vi "Lake Shore 331 Temperature Controller v2.vi"(1 "Loop (0: 1)":u16(ring) items=["1", "2"], 2 "Gain (P)":dbl=50.0 min=0.0 max=1000.0 step=0.1 format="%.1f", 3 "Reset (I)":dbl=50.0 min=0.0 max=1000.0 step=0.1 format="%.1f", 4 "Rate (D)":dbl=100.0 min=0.0 max=200.0 step=1.0, 7 "Manual Output":dbl min=0.0 max=100.0 step=0.001 format="%.3f", 9 "Heater Range (0: Off)":u16(ring)=3 items=["Off", "Low (0.5W)", "Med (5W)", "High (50W)"]) -> (16 "Sensor A":dbl=314.34 min=0.0 max=1645.0 step=1e-05 format="%.5f", 18 "Heater Output":dbl(slide)=100.0 min=0.0 max=100.0 step=0.01 scale=0.0..100.0 scale format="%.1f")   [LabVIEW 2015]
doc: "This VI was designed to demonstrate typical usage of sub vi's containing the more common 331 functions.\n\nThis example configures the loop and setpoint of the instrument, allows for a delay, and then reads sensor and heater output data. The user is given the option of just reading data and not configuring the instrument."
uses:
  <vilib>/Utility/file.llb/Write Delimited Spreadsheet (DBL).vi
  <instrlib>/Lake Shore Cryotronics 331/Lake Shore Cryotronics 331.lvlib
panel:
  in  "Reset":bool
  out "XY Graph":cluster{dbl[], dbl[]}[](graph)=[{array[256 elements], [302.68, 302.68, 302.68, 302.68, 302.68, 302.68, 302.68, 302.68, 302.68, 302.68, 302.68, 302.68, 302.68, 302.68, 302.68, 302.68, 302.68, 302.68, 302.68, 302.68, 302.68, 302.68, 302.68, 302.68, 302.68, 302.68, 302.68, 302.68, 302.68, 302.68, 302.68, 302.68, 302.68, 302.68, 302.68, 302.68, 302.68, 302.68, 302.68, 302.68, 302.68, 302.68, 302.68, 302.68, 302.68, 302.68, 302.68, 302.68, 302.68, 302.68, 302.68, 302.68, 302.68, 302.68, 302.68, 302.68, 302.69, 302.69, 302.69, 302.69, 302.69, 302.69, 302.69, 302.69, 302.7, 302.7, 302.7, 302.7, 302.71, 302.71, 302.72, 302.72, 302.73, 302.73, 302.74, 302.75, 302.76, 302.76, 302.77, 302.78, 302.79, 302.8, 302.82, 302.83, 302.84, 302.85, 302.87, 302.88, 302.9, 302.92, 302.93, 302.95, 302.97, 302.99, 303.01, 303.03, 303.05, 303.08, 303.1, 303.12, 303.15, 303.17, 303.2, 303.23, 303.26, 303.29, 303.32, 303.35, 303.38, 303.41, 303.44, 303.48, 303.51, 303.55, 303.59, 303.62, 303.66, 303.7, 303.74, 303.78, 303.82, 303.86, 303.91, 303.95, 303.99, 304.04, 304.08, 304.13, 304.18, 304.22, 304.27, 304.32, 304.37, 304.42, 304.47, 304.53, 304.58, 304.63, 304.69, 304.74, 304.8, 304.85, 304.91, 304.97, 305.03, 305.09, 305.15, 305.21, 305.27, 305.33, 305.39, 305.45, 305.52, 305.58, 305.64, 305.71, 305.77, 305.84, 305.91, 305.97, 306.04, 306.11, 306.18, 306.25, 306.32, 306.39, 306.46, 306.53, 306.6, 306.67, 306.75, 306.82, 306.89, 306.97, 307.04, 307.12, 307.19, 307.27, 307.34, 307.42, 307.5, 307.58, 307.65, 307.73, 307.81, 307.89, 307.97, 308.05, 308.13, 308.21, 308.3, 308.38, 308.46, 308.54, 308.63, 308.71, 308.79, 308.88, 308.96, 309.05, 309.13, 309.22, 309.3, 309.39, 309.48, 309.56, 309.65, 309.74, 309.82, 309.91, 310.0, 310.09, 310.18, 310.27, 310.36, 310.45, 310.54, 310.63, 310.72, 310.81, 310.9, 310.99, 311.08, 311.18, 311.27, 311.36, 311.45, 311.55, 311.64, 311.73, 311.83, 311.92, 312.02, 312.11, 312.2, 312.3, 312.4, 312.49, 312.59, 312.68, 312.78, 312.88, 312.97, 313.07, 313.17, 313.26, 313.36, 313.46, 313.55, 313.65, 313.75, 313.85, 313.95, 314.04, 314.14, 314.24]}, {array[256 elements], [302.29, 302.29, 302.29, 302.29, 302.29, 302.29, 302.29, 302.29, 302.29, 302.29, 302.29, 302.29, 302.29, 302.29, 302.29, 302.29, 302.29, 302.29, 302.29, 302.29, 302.29, 302.29, 302.29, 302.29, 302.29, 302.29, 302.29, 302.29, 302.29, 302.29, 302.29, 302.29, 302.32, 302.31, 302.31, 302.34, 302.42, 302.56, 302.76, 303.03, 303.34, 303.7, 304.1, 304.52, 304.97, 305.44, 305.93, 306.42, 306.92, 307.42, 307.93, 308.43, 308.93, 309.43, 309.92, 310.41, 310.89, 311.37, 311.83, 312.29, 312.75, 313.19, 313.63, 314.06, 314.48, 314.89, 315.29, 315.69, 316.08, 316.47, 316.84, 317.21, 317.57, 317.93, 318.28, 318.63, 318.96, 319.3, 319.62, 319.94, 320.26, 320.57, 320.87, 321.17, 321.46, 321.75, 322.04, 322.32, 322.6, 322.87, 323.14, 323.41, 323.67, 323.93, 324.18, 324.43, 324.69, 324.93, 325.18, 325.42, 325.66, 325.9, 326.13, 326.36, 326.59, 326.82, 327.04, 327.27, 327.49, 327.71, 327.92, 328.14, 328.35, 328.56, 328.77, 328.98, 329.19, 329.39, 329.6, 329.8, 330.0, 330.2, 330.4, 330.59, 330.79, 330.98, 331.17, 331.37, 331.56, 331.74, 331.93, 332.12, 332.3, 332.49, 332.67, 332.86, 333.04, 333.22, 333.4, 333.58, 333.75, 333.93, 334.11, 334.29, 334.46, 334.64, 334.81, 334.99, 335.16, 335.33, 335.5, 335.67, 335.84, 336.01, 336.18, 336.35, 336.52, 336.69, 336.85, 337.02, 337.18, 337.35, 337.51, 337.68, 337.84, 338.0, 338.17, 338.33, 338.49, 338.65, 338.81, 338.97, 339.13, 339.29, 339.45, 339.61, 339.77, 339.92, 340.08, 340.23, 340.39, 340.54, 340.7, 340.86, 341.01, 341.17, 341.32, 341.47, 341.63, 341.78, 341.93, 342.09, 342.24, 342.39, 342.54, 342.69, 342.85, 343.0, 343.15, 343.27, 343.42, 343.57, 343.72, 343.86, 344.01, 344.16, 344.31, 344.46, 344.61, 344.75, 344.9, 345.05, 345.19, 345.34, 345.49, 345.63, 345.78, 345.92, 346.07, 346.21, 346.36, 346.5, 346.64, 346.78, 346.93, 347.07, 347.21, 347.35, 347.5, 347.64, 347.78, 347.92, 348.06, 348.2, 348.34, 348.48, 348.62, 348.76, 348.9, 349.04, 349.18, 349.32, 349.46, 349.6, 349.74, 349.88, 350.02, 350.15, 350.29, 350.43, 350.57, 350.7, 350.84, 350.98, 351.11, 351.25]}]
  in  "Save":bool
  out "In Range":bool
  in  "Wait Time":dbl=30.0 min=0.0 max=1000.0 step=0.1 format="%.1f"
  in  "Tolerance":dbl=0.1 min=0.0 max=1000.0 step=0.1 format="%.1f"
  in  "Setpoint":dbl=400.0 min=-273.0 max=300000.0 step=0.0001 format="%.4f"
  in  "Control Mode (0: Manual PID)":u16(ring) items=["Manual PID", "Zone", "Open Loop", "AutoTune PID", "AutoTune PI", "AutoTune P"]
  in  "Input to \nControl From":u16(ring)=1 items=["A", "B"]
  out "Loop 1 Heater Range":u16(ring)=3 items=["Off", "Low (0.5W)", "Med (5W)", "High (50W)"]
  out "Manual Output":dbl min=0.0 max=100.0 step=0.001 format="%.3f"
  out "Rate (D)":dbl=100.0 min=0.0 max=1000.0 step=0.1 format="%.1f"
  out "Reset (I)":dbl=50.0 min=0.0 max=1000.0 step=0.1 format="%.1f"
  out "Gain (P)":dbl=50.0 min=0.0 max=1000.0 step=0.1 format="%.1f"
  out "Auto Tuning":bool
  in  "Set":bool
  in  "stop":bool
  out "Waveform Chart":T1(graph)={"Kelvin Reading"=351.25, "Kelvin Reading"=314.24, "Setpoint"=400.0}
  out "Sensor B":dbl=351.25 min=0.0 max=1645.0 step=1e-05 format="%.5f"
  in  "VISA resource name":refnum<visa-resource-name>="COM5"
  # "%"
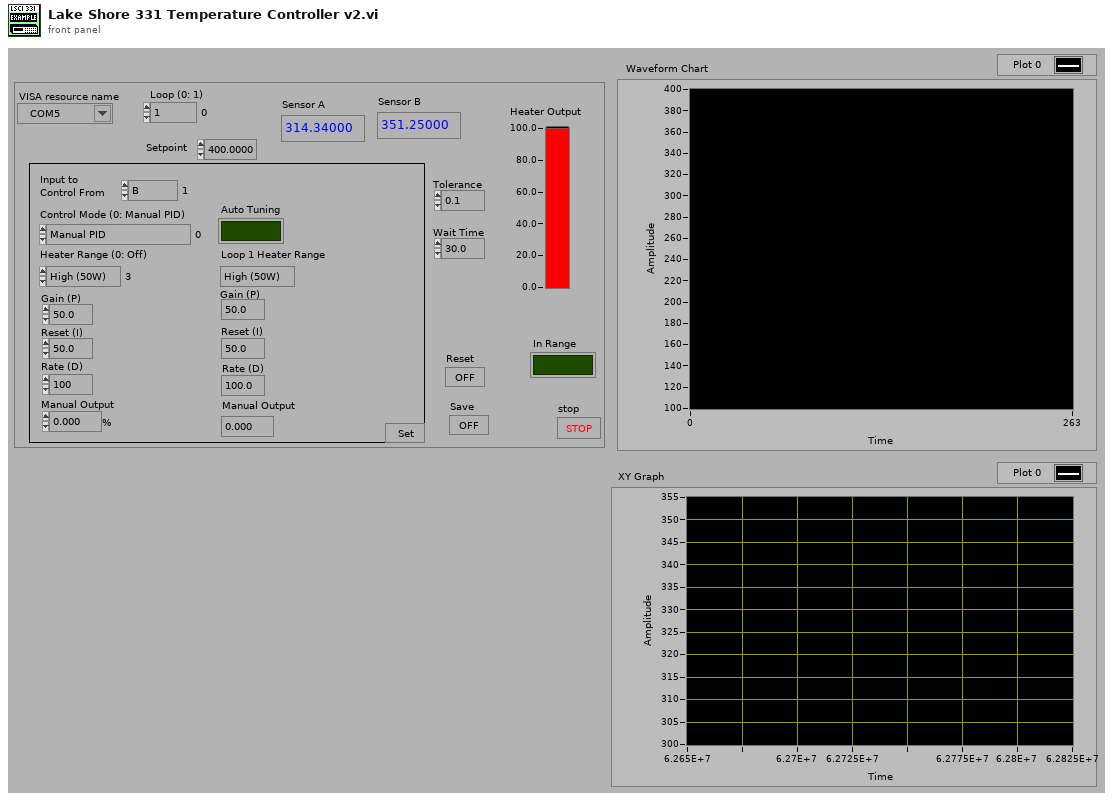
[diagram p1: front panel]
types:
  T1 = cluster{"Kelvin Reading":dbl, "Kelvin Reading":dbl, "Setpoint":dbl}
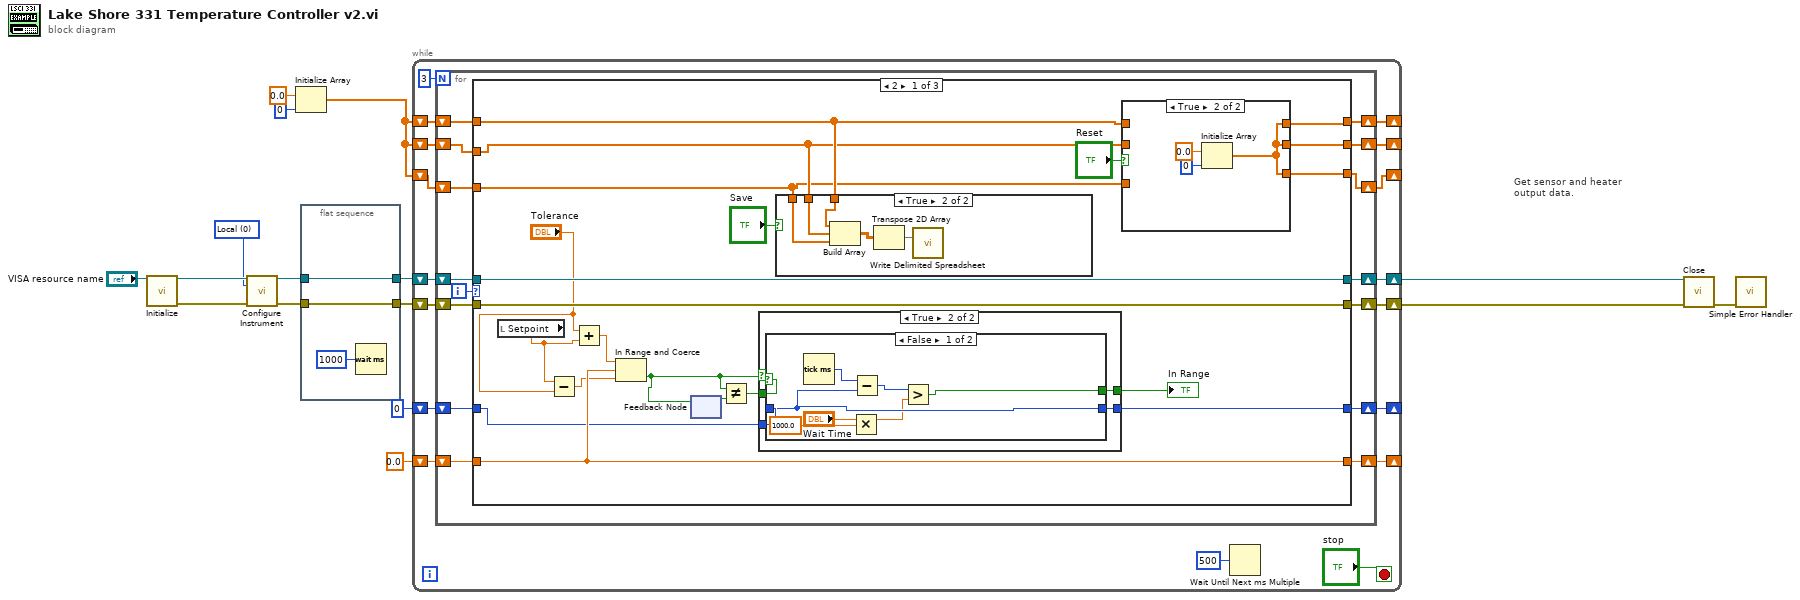
[diagram p0: block diagram]
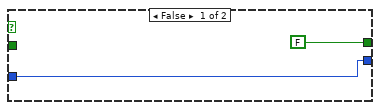
[diagram p4: hidden frame]
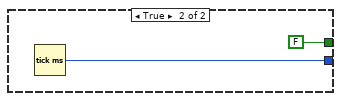
[diagram p5: hidden frame]
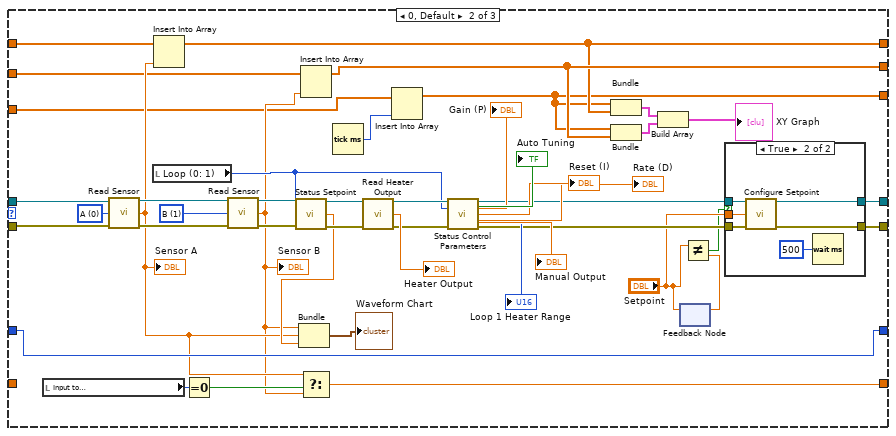
[diagram p6: hidden frame]
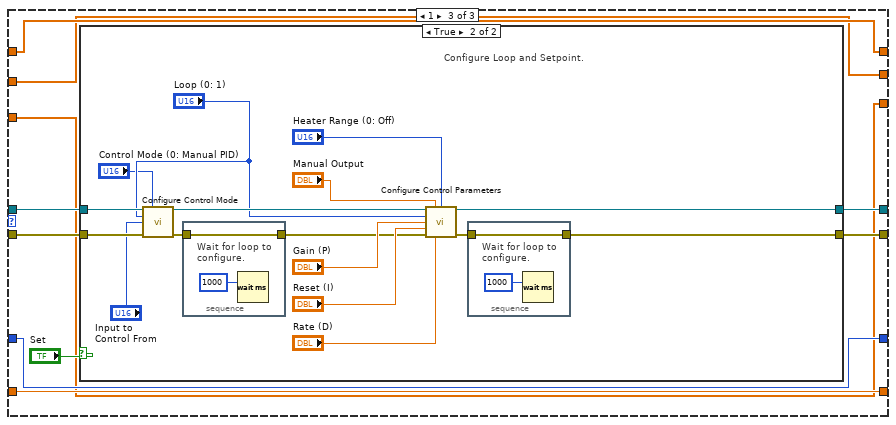
[diagram p8: hidden frame]
diagram:
  w10 = u16 0 items=["Local", "Remote", "Remote w/ Lockout"] ("Remote Interface\nMode (0: Local)")
  # "Get sensor and heater\noutput data."
  n1 = call <instrlib>:"Initialize.vi"("VISA resource name"="VISA resource name") -> ("VISA resource name out"=w12:refnum<visa-resource-name>, "error out"=w11:errorcluster)  [unwired: 13 in]
  n2 = call <instrlib>:"Configure Instrument.vi"("VISA resource name"=w12, "Remote Interface\nMode (0: Local)"=w10, "error in (no error)"=w11) -> ("VISA resource name out"=w9:refnum<visa-resource-name>, "error out"=w7:errorcluster)  [unwired: 11 in]
  n3 = Initialize Array(0.0 ("element"), 0 ("dimension size")) -> (w1:dbl[])
  n4 = flat-sequence {
    tunnel: w9 -> [w19]
    tunnel: [w19] -> w8
    tunnel: w7 -> [w18]
    tunnel: [w18] -> w6
    frame #0 {
      n5 = Wait (ms)(milliseconds to wait=u32 1000) -> ()  [unwired: 1 out]
    }
  }
  n6 = while {
    shift-right: [w34] -> w14
    shift-left: w8 -> [w36]
    shift-right: [w33] -> w13
    shift-left: w6 -> [w35]
    shift-right: [w29] -> _
    shift-left: 0.0 ("Kelvin Reading") -> [w28]
    shift-right: [w27] -> _
    shift-left: u32 0 ("millisecond timer value") -> [w26]
    shift-right: [w22] -> _
    shift-left: w1 -> [w25]
    shift-right: [w23] -> _
    shift-left: w1 -> [w24]
    shift-right: [w20] -> _
    shift-left: w1 -> [w21]
    stop <- "stop" stop-if-true
    n7 = for {
      N: 3 -> [_]
      shift-right: [w49] -> w34
      shift-left: w36 -> [w51]
      shift-right: [w48] -> w33
      shift-left: w35 -> [w50]
      shift-right: [w46] -> w29
      shift-left: w28 -> [w45]
      shift-right: [w44] -> w27
      shift-left: w26 -> [w43]
      shift-right: [w39] -> w22
      shift-left: w25 -> [w42]
      shift-right: [w40] -> w23
      shift-left: w24 -> [w41]
      shift-right: [w37] -> w20
      shift-left: w21 -> [w38]
      i -> [w47]
      n8 = case shown="2" w47 {
        tunnel: w51 -> [w72 w143 w161]
        tunnel: w50 -> [w71 w142 w160]
        tunnel: [w72 w118 w159] -> w49
        tunnel: [w71 w119 w158] -> w48
        tunnel: [w70 w112 w156] -> w46
        tunnel: w45 -> [w70 _ w156]
        tunnel: [w61 w111 w155] -> w44
        tunnel: w43 -> [w60 w111 w155]
        tunnel: w42 -> [w58 w110 w154]
        tunnel: w41 -> [w57 w108 w153]
        tunnel: [w54 w101 w153] -> w40
        tunnel: [w53 w100 w154] -> w39
        tunnel: w38 -> [w56 w106 w152]
        tunnel: [w55 w99 w152] -> w37
        frame 2 {
          n9 = local read "Setpoint"() -> (w68:dbl)
          n10 = Subtract(x=w68, y="Tolerance") -> (x-y=w66:dbl)
          n11 = Add(x="Tolerance", y=w68) -> (x+y=w69:dbl)
          n12 = In Range and Coerce(upper limit=w69, x=w70, lower limit=w66) -> (In Range?=w64:bool)  [unwired: 1 out]
          n13 = feedback #1() -> (w63:bool)  [unwired: 1 in]
          n14 = feedback-in #1(w64) -> ()
          n15 = Not Equal?(x=w64, y=w63) -> (x != y?=w62:bool)
          n16 = case shown="True" w64 {
            tunnel: [FALSE ("In Range") w86] -> w65
            tunnel: w62 -> [_ w89]
            tunnel: [w84 w88] -> w61
            tunnel: w60 -> [w84 w87]
            frame False {
            }
            frame True {
              n17 = case shown="False" w89 {
                tunnel: [w92 w98] -> w88
                tunnel: w87 -> [w92 _]
                tunnel: [w93 FALSE ("In Range")] -> w86
                frame False {
                  n18 = Tick Count (ms)() -> (millisecond timer value=w96:u32)
                  n19 = Multiply(x="Wait Time", y=1000.0) -> (x*y=w91:dbl)
                  n20 = Subtract(x=w96, y=w92) -> (x-y=w95:u32)
                  n21 = Greater?(x=w95, y=w91) -> (0:w93:bool)
                }
                frame True {
                  n22 = Tick Count (ms)() -> (millisecond timer value=w98:u32)
                }
              }
            }
          }
          "In Range" <- w65
          n23 = case shown="True" "Save" {
            tunnel: w58 -> [_ w83]
            tunnel: w57 -> [_ w82]
            tunnel: w56 -> [_ w81]
            frame False {
            }
            frame True {
              n24 = Build Array(w83, w82, w81) -> (w80:dbl[][])
              n25 = Transpose 2D Array(2D array=w80) -> (transposed array=w79:dbl[][])
              n26 = call-poly <vilib>:"Write Delimited Spreadsheet.vi"("2D data"=w79) -> ()  [unwired: 13 in, 2 out]
            }
          }
          n27 = case shown="True" "Reset" {
            tunnel: w58 -> [w73 _]
            tunnel: w57 -> [w74 _]
            tunnel: w56 -> [w75 _]
            tunnel: [w75 w76] -> w55
            tunnel: [w74 w76] -> w54
            tunnel: [w73 w76] -> w53
            frame False {
            }
            frame True {
              n28 = Initialize Array(0.0 ("element"), 0 ("dimension size")) -> (w76:dbl[])
            }
          }
        }
        frame 0, Default {
          w138 = u16 1 items=["A", "B"] ("Input (0: A)")
          w141 = u16 0 items=["A", "B"] ("Input (0: A)")
          n29 = local read "Input to \nControl From"() -> (w114:u16)
          n30 = call <instrlib>:"Read Sensor.vi"("VISA resource name"=w143, "Input (0: A)"=w141, "error in (no error)"=w142) -> ("VISA resource name out"=w140:refnum<visa-resource-name>, "Kelvin Reading"=w109:dbl, "error out"=w139:errorcluster)  [unwired: 8 in, 2 out]
          "Sensor A" <- w109
          n31 = local read "Loop (0: 1)"() -> (w122:u16)
          n32 = Insert Into Array(array=w110, new element=w109) -> (w100:dbl[])  [unwired: 1 in]
          n33 = Equal To 0?(x=w114) -> (x = 0?=w113:bool)
          n34 = call <instrlib>:"Read Sensor.vi"("VISA resource name"=w140, "Input (0: A)"=w138, "error in (no error)"=w139) -> ("VISA resource name out"=w135:refnum<visa-resource-name>, "Kelvin Reading"=w107:dbl, "error out"=w133:errorcluster)  [unwired: 8 in, 2 out]
          "Sensor B" <- w107
          n35 = call <instrlib>:"Status Setpoint.vi"("VISA resource name"=w135, "Loop (0: 1)"=w122, "error in (no error)"=w133) -> ("VISA resource name out"=w134:refnum<visa-resource-name>, "Setpoint"=w131:dbl, "error out"=w132:errorcluster)  [unwired: 10 in]
          n36 = Bundle("Kelvin Reading"=w107, "Kelvin Reading"=w109, "Setpoint"=w131) -> (→"Waveform Chart":T1)  [unwired: 1 in]
          n37 = Insert Into Array(array=w108, new element=w107) -> (w101:dbl[])  [unwired: 1 in]
          n38 = Select(t=w109, s=w113, f=w107) -> (s? t:f=w112:dbl)
          n39 = Tick Count (ms)() -> (millisecond timer value=w105:u32)
          n40 = call <instrlib>:"Read Heater Output.vi"("VISA resource name"=w134, "error in (no error)"=w132) -> ("VISA resource name out"=w130:refnum<visa-resource-name>, "Loop 1\nHeater Output"=→"Heater Output":dbl, "error out"=w129:errorcluster)  [unwired: 11 in]
          n41 = Insert Into Array(array=w106, new element=w105) -> (w99:dbl[])  [unwired: 1 in]
          n42 = call <instrlib>:"Status Control Parameters.vi"("VISA resource name"=w130, "Loop (0: 1)"=w122, "error in (no error)"=w129) -> ("Loop 1 Tuning Status"=→"Auto Tuning":bool, "VISA resource name out"=w121:refnum<visa-resource-name>, "Gain (P)"=→"Gain (P)":dbl, "Reset (I)"=→"Reset (I)":dbl, "Rate (D)"=→"Rate (D)":dbl, "Loop 1 Heater Range"=→"Loop 1 Heater Range":u16, "Manual Output (0.000 %)"=→"Manual Output":dbl, "error out"=w120:errorcluster)  [unwired: 5 in]
          n43 = Bundle(w99, w100) -> (w104:cluster{dbl[], dbl[]})  [unwired: 1 in]
          n44 = Bundle(w99, w101) -> (w103:cluster{dbl[], dbl[]})  [unwired: 1 in]
          n45 = Build Array(w104, w103) -> (→"XY Graph":cluster{dbl[], dbl[]}[])
          n46 = feedback-in #2("Setpoint") -> ()
          n47 = feedback #2() -> (w116:dbl)  [unwired: 1 in]
          n48 = Not Equal?(x="Setpoint", y=w116) -> (x != y?=w115:bool)
          n49 = case shown="True" w115 {
            tunnel: w121 -> [w144 w151]
            tunnel: w120 -> [w145 w150]
            tunnel: [w145 w149] -> w119
            tunnel: [w144 w148] -> w118
            tunnel: "Setpoint" -> [_ w147]
            frame False {
            }
            frame True {
              n50 = call <instrlib>:"Configure Setpoint.vi"("VISA resource name"=w151, "Setpoint (0.0000)"=w147, "error in (no error)"=w150) -> ("VISA resource name out"=w148:refnum<visa-resource-name>, "error out"=w149:errorcluster)  [unwired: 11 in]
              n51 = Wait (ms)(milliseconds to wait=u32 500) -> ()  [unwired: 1 out]
            }
          }
        }
        frame 1 {
          n52 = case shown="True" "Set" {
            tunnel: w160 -> [w162 w171]
            tunnel: w161 -> [w163 w173]
            tunnel: [w162 w166] -> w158
            tunnel: [w163 w167] -> w159
            frame False {
              # "Do not configure Loop and Setpoint."
            }
            frame True {
              # "Configure Loop and Setpoint."
              n53 = call <instrlib>:"Configure Control Mode.vi"("VISA resource name"=w173, "Control Mode (0: Manual PID)"="Control Mode (0: Manual PID)", "Loop (0: 1)"="Loop (0: 1)", "Input to \nControl From (0: A)"="Input to \nControl From", "error in (no error)"=w171) -> ("VISA resource name out"=w172:refnum<visa-resource-name>, "error out"=w165:errorcluster)  [unwired: 9 in]
              n54 = stacked-sequence {
                tunnel: w165 -> [w180]
                tunnel: [w180] -> w164
                frame #0 {
                  # "Wait for loop to \nconfigure."
                  n55 = Wait (ms)(milliseconds to wait=u32 1000) -> ()  [unwired: 1 out]
                }
              }
              n56 = call <instrlib>:"Configure Control Parameters.vi"("VISA resource name"=w172, "Manual Output (0.000 %)"="Manual Output", "Heater Range (0: Off)"="Heater Range (0: Off)", "Loop (0: 1)"="Loop (0: 1)", "Gain (P) (0.0)"="Gain (P)", "Reset (I) (0.0)"="Reset (I)", "error in (no error)"=w164, "Rate (D) (0)"="Rate (D)") -> ("VISA resource name out"=w167:refnum<visa-resource-name>, "error out"=w179:errorcluster)  [unwired: 6 in]
              n57 = stacked-sequence {
                tunnel: w179 -> [w182]
                tunnel: [w182] -> w166
                frame #0 {
                  # "Wait for loop to \nconfigure."
                  n58 = Wait (ms)(milliseconds to wait=u32 1000) -> ()  [unwired: 1 out]
                }
              }
            }
          }
        }
      }
    }
    n59 = Wait Until Next ms Multiple(millisecond multiple=u32 500) -> ()  [unwired: 1 out]
  }
  n60 = call <instrlib>:"Close.vi"("VISA resource name"=w14, "error in (no error)"=w13) -> ("error out"=w16:errorcluster)  [unwired: 13 in]
  n61 = call <vilib>:"Simple Error Handler.vi"("error in (no error)"=w16) -> ()  [unwired: 4 in, 5 out]
